vi "FTW-TransferClient-Upload.vi"(0 "Transfer Client":refnum<class "FTW-TransferClient-S3.lvclass">, 5 "Data":string, 7 "Remote Filename":string, 11 "error in":errorcluster) -> (4 "Transfer Client out":refnum<class "FTW-TransferClient-S3.lvclass">, 6 "URI":string, 8 "Response":string, 10 "Upload Time":u32 format="%06dmsec", 15 "error out":errorcluster)   [LabVIEW 2013, in "FTW-TransferClient-S3.lvclass"]
uses:
  FTW-TransferClient-S3.lvclass
  FTW-TransferClient.lvclass
  FTW-TransferClient-S3.lvclass/FTW-TransferClient-S3.ctl
  C:/Jobs/Tools/featherweight-feature-reorg/source/windows/Transfer Client/S3/AWSSDK.dll
  AWSSDK.dll
panel:
  # "Inputs"
  # "Outputs"
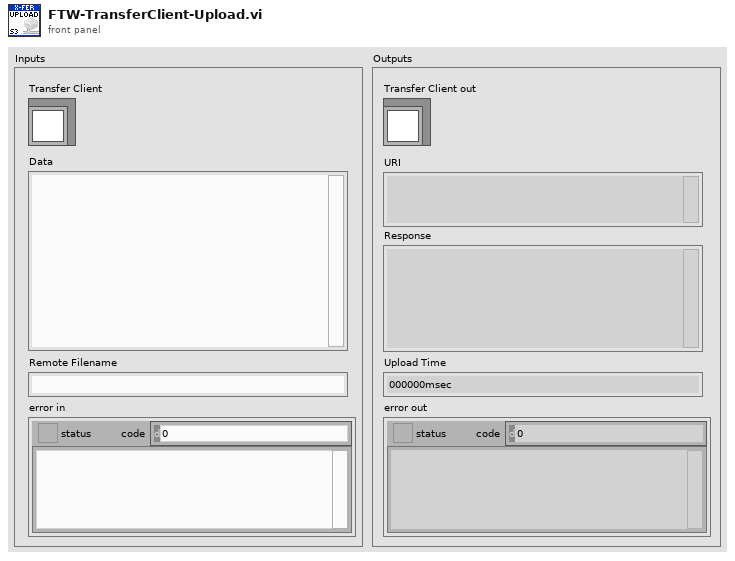
[diagram p1: front panel]
types:
  T1 = typedef "FTW-Collection-KeyValuePair.ctl" = cluster{"Key":string, "Value":string}
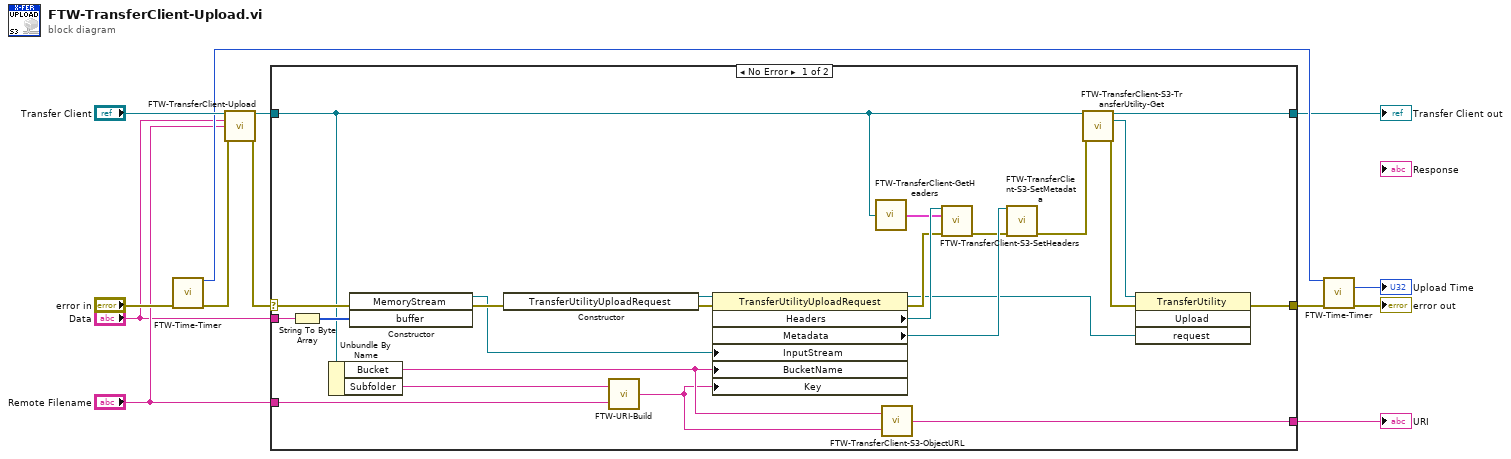
[diagram p0: block diagram]
diagram:
  n1 = call "FTW-Time-Timer.vi"("error in"="error in") -> ("Current Tick Count"=w9:u32, "error out"=w11:errorcluster)  [unwired: 12 in, 1 out]
  n2 = call-parent "FTW-TransferClient-Upload.vi"("Transfer Client"="Transfer Client", "Data"="Data", "Remote Filename"="Remote Filename", "error in"=w11) -> ("Transfer Client out"=w5:refnum<class "FTW-TransferClient-S3.lvclass">, "error out"=w8:errorcluster)  [unwired: 7 in, 3 out]
  n3 = case shown="No Error" w8 {
    selector: w8 -> [w26 w39]
    tunnel: [w28 w39] -> w7
    tunnel: [w30 w38] -> w6
    tunnel: w5 -> [w17 w38]
    tunnel: "Remote Filename" -> [w23 _]
    tunnel: "Data" -> [w22 _]
    tunnel: [w14 _] -> w2
    frame No Error {
      n4 = String To Byte Array(string=w22) -> (unsigned byte array=w21:u8[])
      n5 = Unbundle By Name(w17) -> ("Bucket"=w16:string, "Subfolder"=w27:string)
      n6 = constructor class="MemoryStream"(error in=w26, "buffer"=w21) -> (reference out=w24:refnum<k24>, error out=w25:errorcluster)  [unwired: 2 in, 2 out]
      n7 = constructor class="TransferUtilityUploadRequest"(error in=w25) -> (reference out=w37:refnum<k24>, error out=w36:errorcluster)  [unwired: 2 in, 1 out]
      n8 = call "FTW-URI-Build.vi"("Base URI"=w27, "Relative URI"=w23) -> ("Output"=w15:string)  [unwired: 3 in]
      n9 = property class="TransferUtilityUploadRequest"(reference=w37, error in=w36, "InputStream"=w24, "BucketName"=w16, "Key"=w15) -> (reference out=w31:refnum<k24>, error out=w33:errorcluster, "Headers"=w35:refnum<k24>, "Metadata"=w34:refnum<k24>)
      n10 = call "FTW-TransferClient-GetHeaders.vi"("Transfer Client"=w17) -> ("Headers"=w18:T1[])
      n11 = call "FTW-TransferClient-S3-ObjectURL.vi"("Object Bucket"=w16, "Object Key"=w15) -> ("Object URL"=w14:string)  [unwired: 2 in]
      n12 = call "FTW-TransferClient-S3-SetHeaders.vi"("Headers"=w35, "Headers Collection"=w18, "error in"=w33) -> ("error out"=w32:errorcluster)  [unwired: 12 in]
      n13 = call "FTW-TransferClient-S3-SetMetadata.vi"("Metadata"=w34, "error in"=w32) -> ("error out"=w20:errorcluster)  [unwired: 13 in]
      n14 = call "FTW-TransferClient-S3-TransferUtility-Get.vi"("Transfer Client"=w17, "error in"=w20) -> ("Transfer Client out"=w30:refnum<class "FTW-TransferClient-S3.lvclass">, "Transfer Utility ref"=w29:refnum<k24>, "error out"=w19:errorcluster)  [unwired: 11 in]
      n15 = invoke class="TransferUtility" method="Upload"(reference=w29, error in=w19, "request"=w31) -> (error out=w28:errorcluster)  [unwired: 1 in, 3 out]
    }
    frame Error {
    }
  }
  "Transfer Client out" <- w6
  "URI" <- w2
  n16 = call "FTW-Time-Timer.vi"("Initial Tick Count"=w9, "error in"=w7) -> ("Elapsed Time"=→"Upload Time":u32, "error out"=→"error out":errorcluster)  [unwired: 11 in, 1 out]
